vi "Add Fruit Class.vi"(8 "error in (no error)":errorcluster, 10 "Fruit":refnum<class "Fruit.lvclass">, 11 "Board_Game in":refnum<class "Board_Game.lvclass">) -> (0 "error out":errorcluster, 3 "Board_Game out":refnum<class "Board_Game.lvclass">)   [LabVIEW 2021, in "Board_Game.lvclass"]
uses:
  Board_Game.lvclass
  Fruit/Fruit.lvclass
  Board_Game.lvclass/Board_Game.ctl
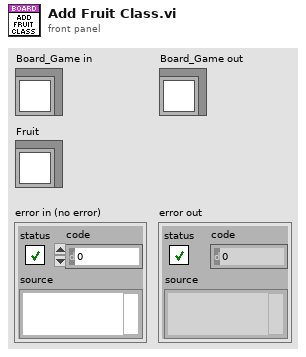
[diagram p1: front panel]
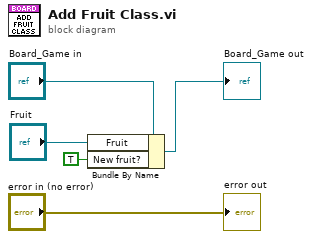
[diagram p0: block diagram]
diagram:
  n1 = Bundle By Name(cluster="Board_Game in", "Fruit"="Fruit", "New fruit?"=TRUE) -> (→"Board_Game out":refnum<class "Board_Game.lvclass">)
  "error out" <- "error in (no error)"
